vi "Demo Init.vi"() -> (14 "Colleague Array":refnum<class "Device.lvclass">[](array[class]), 15 "Output":string, 19 "错误输出":errorcluster)   [LabVIEW 2013]
uses:
  Device_class/Device.lvclass
  Mediator_class/Mediator.lvclass
  Colleague_class/Colleague.lvclass
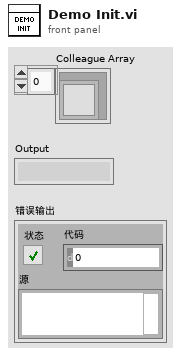
[diagram p1: front panel]
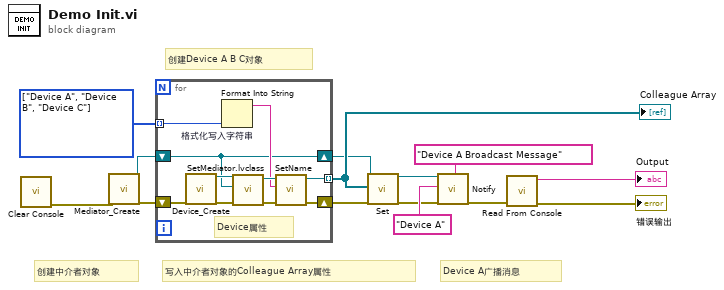
[diagram p0: block diagram]
diagram:
  w3 = enum16{"Device A", "Device B", "Device C"}[] [enum."Device A", enum."Device B", enum."Device C"] items=["Device A", "Device B", "Device C"]
  # "创建Device A B C对象"
  # "Device A广播消息"
  # "写入中介者对象的Colleague Array属性"
  # "创建中介者对象"
  n1 = call "Clear Console.vi"() -> ("error out"=w6:errorcluster)  [unwired: 11 in]
  n2 = call "Mediator_Create.vi"("error in (no error)"=w6) -> ("reference out"=w5:refnum<class "Mediator.lvclass">, "error out"=w2:errorcluster)  [unwired: 17 in]
  n3 = for {
    tunnel: w3 -> [w22] mode=indexing
    tunnel: [w20] -> w10 mode=indexing
    shift-right: [w19] -> w4
    shift-left: w2 -> [w18]
    shift-right: [w15] -> w1
    shift-left: w5 -> [w15]
    # "Device属性"
    n4 = call "Device_Create.vi"("error in (no error)"=w18) -> ("reference out"=w16:refnum<class "Device.lvclass">, "error out"=w17:errorcluster)  [unwired: 17 in]
    n5 = Format Into String "格式化写入字符串"(w22) -> (resulting string=w21:string)  [unwired: 3 in, 1 out]
    n6 = call "SetMediator.lvclass.vi"("error in (no error)"=w17, "Mediator.lvclass"=w15, "reference in"=w16) -> ("error out"=w24:errorcluster, "reference out"=w23:refnum<class "Device.lvclass">)  [unwired: 7 in]
    n7 = call "SetName.vi"("error in (no error)"=w24, "Name"=w21, "reference in"=w23) -> ("error out"=w19:errorcluster, "reference out"=w20:refnum<class "Device.lvclass">)  [unwired: 7 in]
  }
  "Colleague Array" <- w10
  n8 = call "Set.vi"("reference in"=w1, "Colleague"=w10, "error in (no error)"=w4) -> ("reference out"=w11:refnum<class "Mediator.lvclass">, "error out"=w7:errorcluster)  [unwired: 15 in]
  n9 = call-dynamic "Notify.vi"("reference in"=w11, "Sender"="Device A", "error in (no error)"=w7, "Message"="Device A Broadcast Message") -> ("error out"=w12:errorcluster)  [unwired: 14 in, 1 out]
  n10 = call "Read From Console.vi"("error in (no error)"=w12) -> ("error out"=→"错误输出":errorcluster, "Output"=→"Output":string)  [unwired: 9 in]
